vi "Bring Window Forward (WinAPI).vi"(8 "error in (no error)":errorcluster, 11 "VI reference in":refnum<vi>) -> (0 "error out":errorcluster, 1 "Handle":u64, 3 "VI reference out":refnum<vi>)   [LabVIEW 2017]
uses:
  USER32.DLL
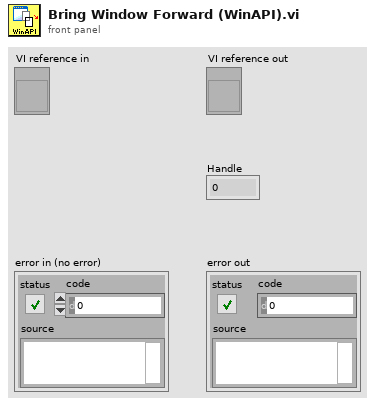
[diagram p1: front panel]
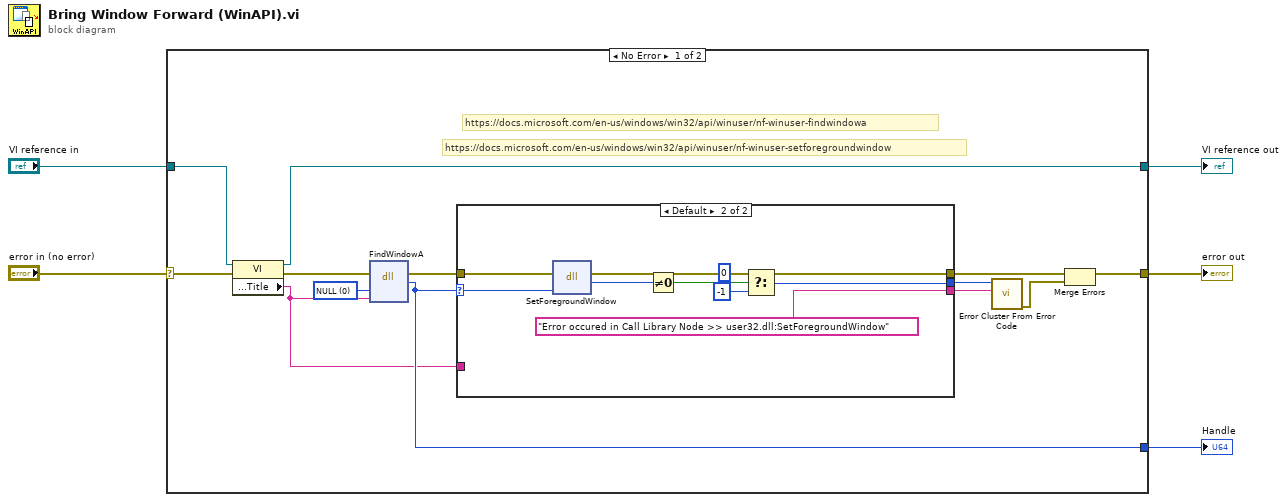
[diagram p0: block diagram]
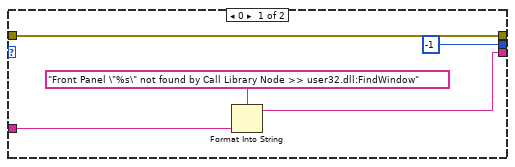
[diagram p2: hidden frame]
diagram:
  n1 = case shown="No Error" "error in (no error)" {
    selector: "error in (no error)" -> [w12 w34]
    tunnel: [w11 w34] -> w5
    tunnel: [w10 _] -> w4
    tunnel: [w14 w33] -> w3
    tunnel: "VI reference in" -> [w13 w33]
    frame No Error {
      w16 = 0 items=["NULL"]
      # "https://docs.microsoft.com/en-us/windows/win32/api/winuser/nf-winuser-findwindowa"
      # "https://docs.microsoft.com/en-us/windows/win32/api/winuser/nf-winuser-setforegroundwindow"
      n2 = property class="VI"(reference=w13, error in=w12) -> (reference out=w14:refnum<vi>, error out=w15:errorcluster, "Front Panel.Title"=w6:string)
      n3 = dll-call lib="user32.dll" fn="FindWindowA"(error in=w15, "lpszClassName"=w16, "lpszWindowName"=w6) -> (error out=w17:errorcluster, "hWnd"=w10:u64)  [unwired: 3 in, 2 out]
      n4 = case shown="Default" w10 {
        selector: w10 -> [_ w29]
        tunnel: [w23 w32] -> w18
        tunnel: w17 -> [w23 w31]
        tunnel: [-1 ("return type") w27] -> w8
        tunnel: [w20 "Error occured in Call Library Node >> user32.dll:SetForegroundWindow" ("error message (\"\")")] -> w7
        tunnel: w6 -> [w19 _]
        frame 0 {
          n5 = Format Into String(format string="Front Panel \"%s\" not found by Call Library Node >> user32.dll:FindWindow" ("error message (\"\")"), w19) -> (resulting string=w20:string)  [unwired: 2 in, 1 out]
        }
        frame Default {
          n6 = dll-call lib="USER32.DLL" fn="SetForegroundWindow"(error in=w31, "Handle"=w29) -> (error out=w32:errorcluster, "return type"=w26:i32)  [unwired: 3 in, 1 out]
          n7 = Not Equal To 0?(x=w26) -> (x != 0?=w28:bool)
          n8 = Select(t=0, s=w28, f=-1) -> (s? t:f=w27:i32)
        }
      }
      n9 = call <vilib>:"Error Cluster From Error Code.vi"("error message (\"\")"=w7, "error code (0)"=w8) -> ("error out"=w9:errorcluster)  [unwired: 7 in]
      n10 = Merge Errors(w18, w9) -> (w11:errorcluster)
    }
    frame Error {
    }
  }
  "Handle" <- w4
  "error out" <- w5
  "VI reference out" <- w3
